vi "Set Transfer Group Parameters.vi"(10 "Transfer Group parameters":T1[](array[typedef]) {"Rx"."max size" format="%d bytes"; "Rx"."Transfers Rx"."source address" format="%d ms"; "Rx"."Transfers Rx"."timeout" format="%d bytes"}, 11 "UDP Transceiver in":refnum<class "UDP Transceiver.lvclass">) -> (3 "UDP Transceiver out":refnum<class "UDP Transceiver.lvclass">)   [LabVIEW 2017, in "UDP Transceiver.lvlib" / "UDP Transceiver.lvclass"]
uses:
  UDP Transceiver.lvclass
  UDP Transfer Group Parameters.ctl
  UDP Transfer Group Receive Parameters.ctl
  UDP Transfer Receive Parameters.ctl
  UDP Transfer Group Transmit Parameters.ctl
  UDP Transfer Transmit Parameters.ctl
  UDP Transceiver.lvclass/UDP Transceiver.ctl
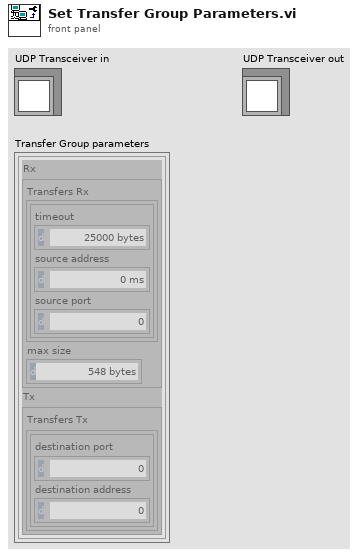
[diagram p1: front panel]
types:
  T1 = typedef "UDP Transceiver.lvlib/UDP Transceiver.lvclass/UDP Transfer Group Parameters.ctl" = cluster{"Rx":T2, "Tx":T4}
  T2 = typedef "UDP Transceiver.lvlib/UDP Transceiver.lvclass/UDP Transfer Group Receive Parameters.ctl" = cluster{"Transfers Rx":T3[], "max size":i32}
  T3 = typedef "UDP Transceiver.lvlib/UDP Transceiver.lvclass/UDP Transfer Receive Parameters.ctl" = cluster{"timeout":i32, "source address":u32, "source port":u16}
  T4 = typedef "UDP Transceiver.lvlib/UDP Transceiver.lvclass/UDP Transfer Group Transmit Parameters.ctl" = cluster{"Transfers Tx":T5[]}
  T5 = typedef "UDP Transceiver.lvlib/UDP Transceiver.lvclass/UDP Transfer Transmit Parameters.ctl" = cluster{"destination port":u16, "destination address":u32}
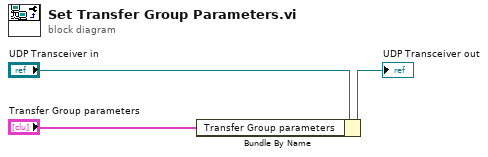
[diagram p0: block diagram]
diagram:
  n1 = Bundle By Name(cluster="UDP Transceiver in", "Transfer Group parameters"="Transfer Group parameters") -> (→"UDP Transceiver out":refnum<class "UDP Transceiver.lvclass">)
